vi "状态读取.vi"(7 "运行模式":string, 8 "error in (no error)":errorcluster, 11 "Slave ID":T4) -> (0 "error out":errorcluster, 2 "质控仪器状态显示":T1, 3 "质控仪器状态":T2)   [LabVIEW 2016, in "质控单元V1.lvlib"]
uses:
  <vilib>/Plasmionique/MB Master/MB_Master/MB_Master.lvclass
  <vilib>/Plasmionique/MB Master/MB Master.lvlib
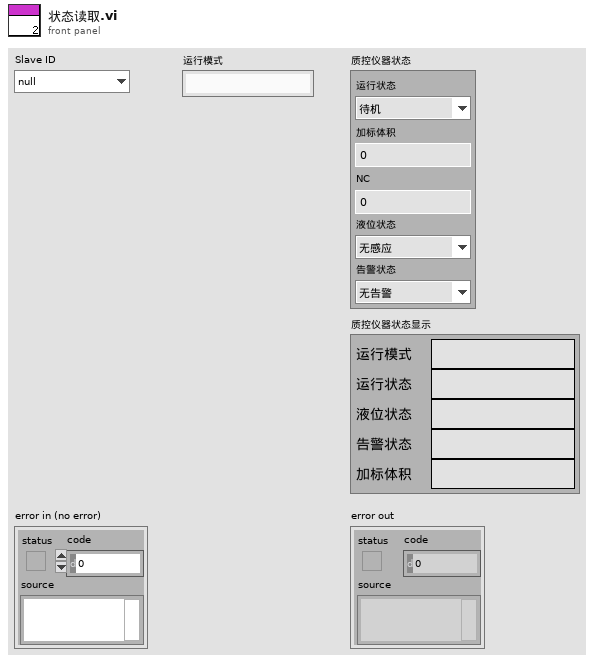
[diagram p1: front panel]
types:
  T1 = typedef "质控单元V1.lvlib/质控仪器状态显示.ctl" = cluster{"运行模式":string, "运行状态":string, "液位状态":string, "告警状态":string, "加标体积":string}
  T2 = typedef "质控单元V1.lvlib/质控仪器状态.ctl" = cluster{"运行状态":T3, "加标体积":sgl, "NC":dbl, "液位状态":enum16{"无感应", "有感应"}, "告警状态":enum16{"无告警", "超时告警"}}
  T3 = typedef "质控单元V1.lvlib/质控运行状态.ctl" = enum16{"待机", "润洗", "进样", "加标", "排液", "搅拌", "超时告警"}
  T4 = typedef "质控单元V1.lvlib/质控slave id.ctl" = enum16{"null", "氨氮", "总磷", "CODMn", "CODCr", "总氮"}
  T5 = cluster{"Registers[0]":u16, "Registers[1]":u16, "Registers[2]":u16, "Registers[3]":u16, "Registers[4]":u16}
  T6 = cluster{"运行模式":string, "RingText.Text":string, "RingText.Text":string, "RingText.Text":string, "NumText.Text":string}
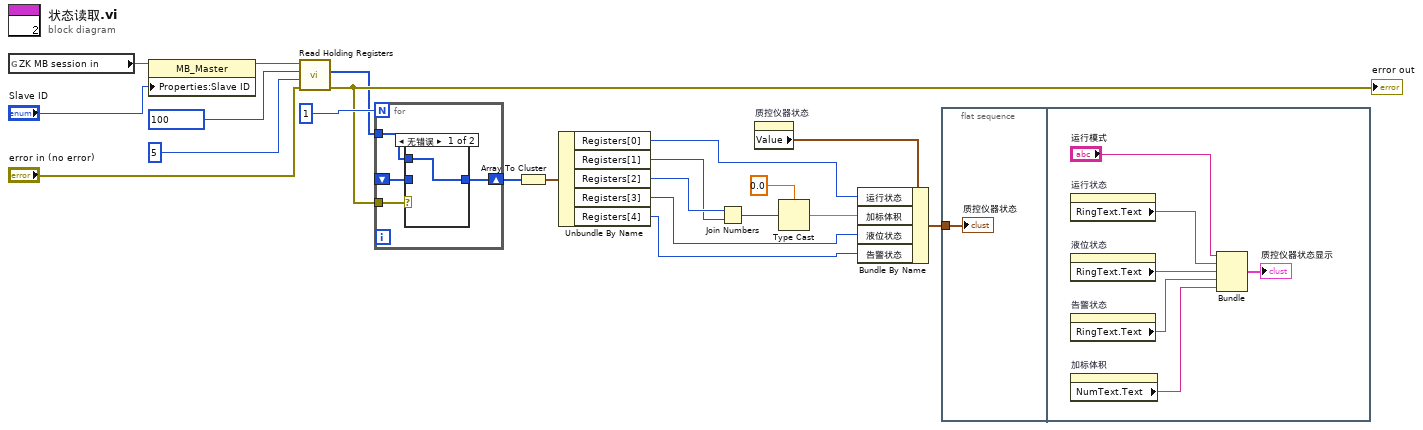
[diagram p0: block diagram]
diagram:
  n1 = global read "ZK非断电保存全局变量.vi" "ZK MB session in"() -> (w20:refnum<class "MB_Master.lvclass">)
  n2 = property class="MB_Master"(reference=w20, "Properties:Slave ID"="Slave ID") -> (reference out=w18:refnum<class "MB_Master.lvclass">)  [unwired: 1 in, 1 out]
  n3 = call <vilib>:"Read Holding Registers.vi"("error in (no error)"="error in (no error)", "quantity"=u16 5, "starting address"=u16 100, "MB session in"=w18) -> ("error out"=w15:errorcluster, "Registers"=w14:u16[])  [unwired: 5 in, 1 out]
  "error out" <- w15
  n4 = for {
    N: 1 -> [_]
    tunnel: w15 -> [w25]
    tunnel: w14 -> [w24]
    shift-right: [w23] -> w1
    shift-left: _ -> [w22]
    n5 = case shown="无错误" w25 {
      tunnel: w24 -> [w26 _]
      tunnel: [w26 w27] -> w23
      tunnel: w22 -> [_ w27]
      frame No Error {
      }
      frame Error {
      }
    }
  }
  n6 = Array To Cluster(array=w1) -> (cluster=w8:T5)
  n7 = Unbundle By Name(w8) -> ("Registers[0]"=w4:u16, "Registers[1]"=w11:u16, "Registers[2]"=w12:u16, "Registers[3]"=w3:u16, "Registers[4]"=w2:u16)
  n8 = Join Numbers(hi=w12, lo=w11) -> ((hi.lo)=w10:u32)
  n9 = property on="质控仪器状态" class="Clust (严格)"() -> ("Value"=w7:T2)  [unwired: 2 in, 2 out]
  n10 = Type Cast(type=sgl 0.0, x=w10) -> (*(type *) &x=w5:sgl)
  n11 = Bundle By Name(cluster=w7, "运行状态"=w4, "加标体积"=w5, "液位状态"=w3, "告警状态"=w2) -> (w6:T2)
  n12 = flat-sequence {
    tunnel: w6 -> [w28]
    frame #0 {
      "质控仪器状态" <- w28
    }
    frame #1 {
      n13 = property on="运行状态" class="Enum (严格)"() -> ("RingText.Text"=w34:string)  [unwired: 2 in, 2 out]
      n14 = property on="液位状态" class="Enum (严格)"() -> ("RingText.Text"=w31:string)  [unwired: 2 in, 2 out]
      n15 = property on="告警状态" class="Enum (严格)"() -> ("RingText.Text"=w29:string)  [unwired: 2 in, 2 out]
      n16 = property on="加标体积" class="DigNum (严格)"() -> ("NumText.Text"=w30:string)  [unwired: 2 in, 2 out]
      n17 = Bundle("运行模式"="运行模式", "RingText.Text"=w34, "RingText.Text"=w31, "RingText.Text"=w29, "NumText.Text"=w30) -> (→"质控仪器状态显示":T6)  [unwired: 1 in]
    }
  }
